vi "isSharedResource.vi"(8 "error in (no error)":errorcluster, 11 "SMO in":refnum<class "SMO.lvclass">) -> (0 "error out":errorcluster, 2 "shared resource":bool, 3 "SMO out":refnum<class "SMO.lvclass">)   [LabVIEW 2013, in "SMO.lvclass"]
uses:
  SMO.lvclass
  Support/Attribute.SharedResource/Attribute.SharedResource.lvclass
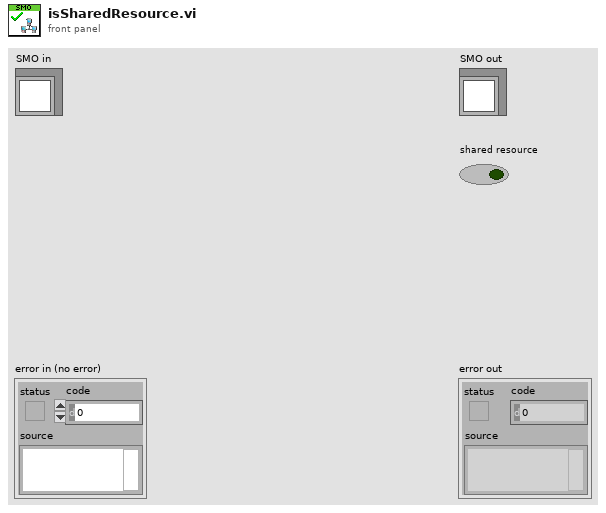
[diagram p1: front panel]
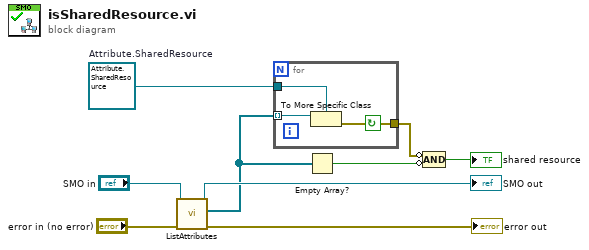
[diagram p0: block diagram]
diagram:
  w6 = refnum<class "Attribute.SharedResource.lvclass"> refnum  # Attribute.SharedResource
  n1 = call "ListAttributes.vi"("error in (no error)"="error in (no error)", "SMO in"="SMO in") -> ("error out"=→"error out":errorcluster, "[Attributes]"=w4:refnum<class "Attribute.lvclass">[], "SMO out"=→"SMO out":refnum<class "SMO.lvclass">)  [unwired: 7 in]
  n2 = for {
    tunnel: w4 -> [w12] mode=indexing
    tunnel: w6 -> [w11]
    tunnel: [w10] -> w2
    stop <- w10 continue-if-true
    n3 = To More Specific Class(target class=w11, reference=w12) -> (error out=w10:errorcluster)  [unwired: 1 in, 1 out]
  }
  n4 = Empty Array?(array=w4) -> (empty?=w3:bool)
  n5 = Compound Arithmetic op=AND(invert w2, invert w3) -> (→"shared resource":bool)
